vi "Revision Management.vi"() -> (2 "Software Revision Number":string)   [LabVIEW 2013]
uses:
  Typedefs/Which path.ctl
  Global Variables/General Globals.vi
  <vilib>/Utility/config.llb/Read Key (String).vi
  <vilib>/Utility/config.llb/Write Key (String).vi
  Global Variables/gl_UI Ctrl Refs.vi
  <vilib>/Utility/config.llb/NI_LVConfig.lvlib
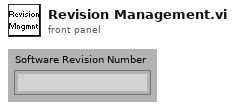
[diagram p1: front panel]
types:
  T1 = typedef "Which path.ctl" = enum16{"Configuration Files", "Calibration Files", "Images", "Setup.ini", "Loaded User profile.ini", "User's-Previous session.ini", "New user profile.ini", "Selected User profile.ini", "User profiles folder", "Power meter scaling.txt", "FOV Cal.ini"}
  T2 = enum32{"invalid app kind", "Development System", "Run Time System", "Student Edition", "Embedded LabVIEW", "Evaluation", "Custom"}
  T3 = typedef "NI_LVConfig.lvlib/Config Data RefNum.ctl" = refnum<k1>
  T4 = typedef "UI ctrl refs cluster.ctl" = cluster{"Top level VI path":path, "Top level VI ref":refnum<vi>, "User menu ref":refnum<k9>, "Sub Panel control":refnum<vi>, "Imaging Param Tab":refnum<vi>, "Occurrence-Start drivers":refnum<k4>, "Occurrence-Speed logging initialised":refnum<k4>, "Occurrence-XYZ stage initialised":refnum<k4>, "Exit button":refnum<vi>, "Status ind":refnum<vi>, "Return to Origin":refnum<vi>, "Speed Logging":refnum<vi>, "Time Lapse":refnum<vi>, "Live Imaging":refnum<vi>, "AOL Z Stack":refnum<vi>, "Motor Z Stack":refnum<vi>, "Funct Acq button":refnum<vi>, "Hard Shutter":refnum<vi>, "Virtual Shutter":refnum<vi>, "Laser Power":refnum<vi>, "AOL Mode":refnum<vi>, "Frame Size":refnum<vi>, "Field of View":refnum<vi>, "Dwell Time":refnum<vi>, "Zoom":refnum<vi>, "AOL Z":refnum<vi>, "Objective":refnum<vi>, "Axis":refnum<vi>, "Paths & Names":refnum<vi>, "Experiment folder path (ind.)":refnum<vi>, "Last State (Ind.)":refnum<vi>, "Laser wavelength ind (nm)":refnum<vi>, "Averages":refnum<vi>, "Angle (degrees)":refnum<vi>, "X centre":refnum<vi>, "Y centre":refnum<vi>, "Plane Mode":refnum<vi>, "# Planes":refnum<vi>, "Z Start":refnum<vi>, "Z Stop":refnum<vi>, "Z Step":refnum<vi>, "PMT 1":refnum<vi>, "PMT 2":refnum<vi>, "Stage XYZ Position":refnum<vi>, "Pockels@Z Start":refnum<vi>, "Pockels@Z Stop":refnum<vi>, "Obtain Z Start":refnum<vi>, "Obtain Z Stop":refnum<vi>, "Live stim.trig.period":refnum<vi>, "Live stim.trig.enable":refnum<vi>, "Funct. Acq. Pockels Modulation":refnum<vi>, "Enable Video Recording":refnum<vi>, "Video Record-Live Imaging":refnum<vi>, "Video Record-Funct acq":refnum<vi>, "AOL Z-stack Chirps Ready (ind)":refnum<vi>, "Center freq ind (nm)":refnum<vi>, "Logging queue (ind)":refnum<vi>, "Back aperture power (ind.)":refnum<vi>, "Power after objective (ind.)":refnum<vi>, "Switch user":refnum<vi>}
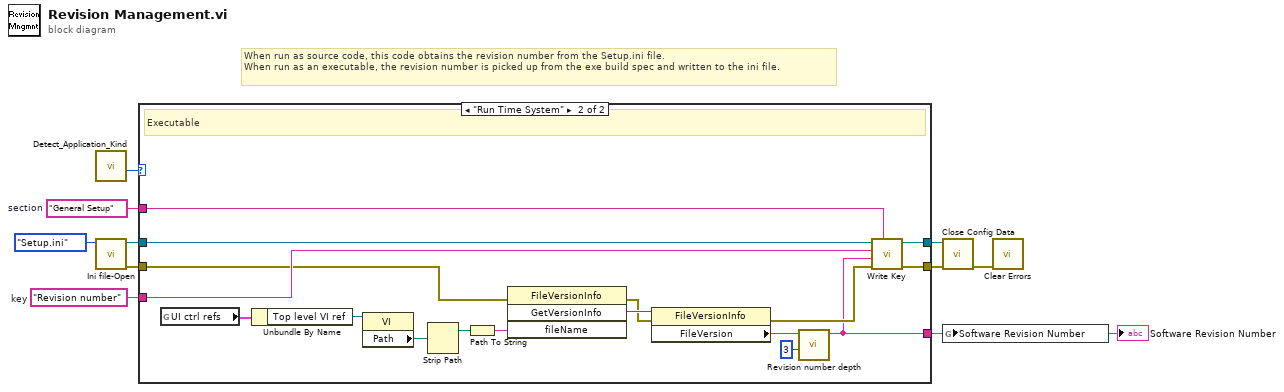
[diagram p0: block diagram]
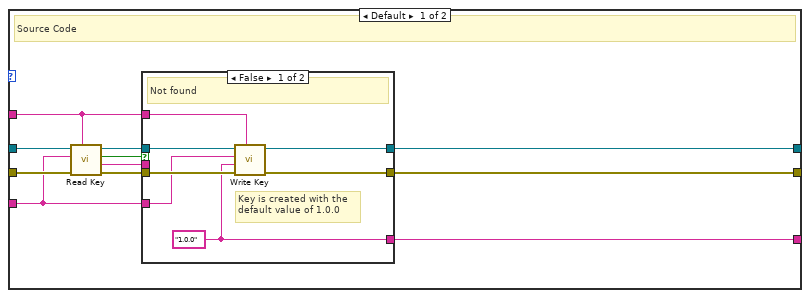
[diagram p2: hidden frame]
diagram:
  w8 = "Revision number"  # key
  w9 = "General Setup"  # section
  # "When run as source code, this code obtains the revision number from the Setup.ini file.\nWhen run as an executable, the revision number is picked up from the exe build spec and written to the ini file."
  n1 = call "Detect_Application_Kind.vi"() -> ("Application:Kind"=w10:T2)  [unwired: 9 in, 2 out]
  n2 = call "Ini file-Open.vi"("Which file?"=Which_path."Setup.ini") -> ("error out"=w4:errorcluster, "User profile ini file ref"=w5:T3)  [unwired: 7 in, 2 out]
  n3 = case shown="\"Run Time System\"" w10 {
    tunnel: [w17 w39] -> w7
    tunnel: w5 -> [w20 w44]
    tunnel: w9 -> [w14 w43]
    tunnel: w8 -> [w13 w42]
    tunnel: w4 -> [w21 w34]
    tunnel: [w12 w33] -> w2
    tunnel: [w11 w32] -> w3
    frame Default {
      # "Source Code"
      n4 = call-poly <vilib>:"Read Key.vi"("section"=w14, "error in (no error)"=w21, "key"=w13, "refnum"=w20) -> ("error out"=w15:errorcluster, "value"=w18:string, "found?"=w19:bool, "refnum out"=w16:T3)  [unwired: 4 in]
      n5 = case shown="False" w19 {
        tunnel: w18 -> [_ w31]
        tunnel: [w24 w31] -> w17
        tunnel: w16 -> [w28 w29]
        tunnel: w15 -> [w27 w30]
        tunnel: w14 -> [w26 _]
        tunnel: w13 -> [w25 _]
        tunnel: [w23 w30] -> w11
        tunnel: [w22 w29] -> w12
        frame False {
          w24 = "1.0.0" ("value")
          # "Key is created with the \ndefault value of 1.0.0"
          # "Not found"
          n6 = call-poly <vilib>:"Write Key.vi"("section"=w26, "error in (no error)"=w27, "value"=w24, "key"=w25, "refnum"=w28) -> ("error out"=w23:errorcluster, "refnum out"=w22:T3)  [unwired: 4 in, 1 out]
        }
        frame True {
          # "Found"
        }
      }
    }
    frame "Run Time System" {
      # "Executable"
      n7 = global read "gl_UI Ctrl Refs.vi" "UI ctrl refs"() -> (w37:T4)
      n8 = Unbundle By Name(w37) -> ("Top level VI ref"=w38:refnum<vi>)
      n9 = property class="VI"(reference=w38) -> ("Path"=w36:path)  [unwired: 1 in, 2 out]
      n10 = Strip Path(path=w36) -> (stripped path=w46:path)  [unwired: 1 out]
      n11 = Path To String(path=w46) -> (string=w48:string)
      n12 = invoke class="FileVersionInfo" method="GetVersionInfo"(error in=w34, "fileName"=w48) -> (error out=w45:errorcluster, "GetVersionInfo"=w47:refnum<k24>)  [unwired: 2 in, 2 out]
      n13 = property class="FileVersionInfo"(reference=w47, error in=w45) -> (error out=w41:errorcluster, "FileVersion"=w40:string)  [unwired: 1 out]
      n14 = call "Revision number depth.vi"("Depth (2)"=u8 3, "Full software Revision Number"=w40) -> ("Software Revision Number (first 2 levels only)"=w39:string)  [unwired: 9 in]
      n15 = call-poly <vilib>:"Write Key.vi"("section"=w43, "error in (no error)"=w41, "value"=w39, "key"=w42, "refnum"=w44) -> ("error out"=w32:errorcluster, "refnum out"=w33:T3)  [unwired: 4 in, 1 out]
    }
  }
  "Software Revision Number" <- w7
  n16 = call <vilib>:"Close Config Data.vi"("error in (no error)"=w3, "refnum"=w2) -> ("error out"=w1:errorcluster)  [unwired: 8 in, 1 out]
  n17 = global write "General Globals.vi" "Software Revision Number"(w7) -> ()
  n18 = call <vilib>:"Clear Errors.vi"("error in (no error)"=w1) -> ()  [unwired: 6 in, 1 out]
